vi "Main_UI.vi"() -> ()   [LabVIEW 2015]
uses:
  utilities/GlobalSender.vi
panel:
  out "GAS":bool
  out "BRAKES":bool
  in  "stop":bool
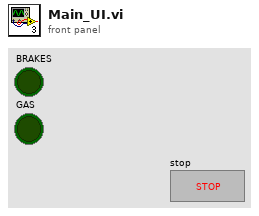
[diagram p1: front panel]
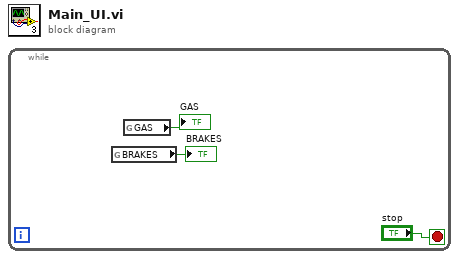
[diagram p0: block diagram]
diagram:
  n1 = while {
    stop <- "stop" stop-if-true
    n2 = global read "GlobalSender.vi" "BRAKES"() -> (→"BRAKES":bool)
    n3 = global read "GlobalSender.vi" "GAS"() -> (→"GAS":bool)
  }
